vi "Take_photo.vi"(7 "error in":errorcluster, 10 "Session In":T3) -> (0 "error out":errorcluster, 2 "x = y?":bool)   [LabVIEW 2020]
doc: "Take photo if matching template."
uses:
  <vilib>/userDefined/High Color/IMAQdx.ctl
  <vilib>/vision/driver/NI_Vision_Acquisition_Software.lvlib
  <vilib>/vision/NI_Vision_Development_Module.lvlib
panel:
  out "Application Directory 3":path
  out "Application Directory 2":path
  out "Number of Matches":i32
  out "Image 2":T1(plugin-control)
  in  "Parameters":T2={"Number of Matches Requested"=1, "Minimum Match Score"=800.0, "Angle Ranges"=[]}
  out "Image":T1(plugin-control)
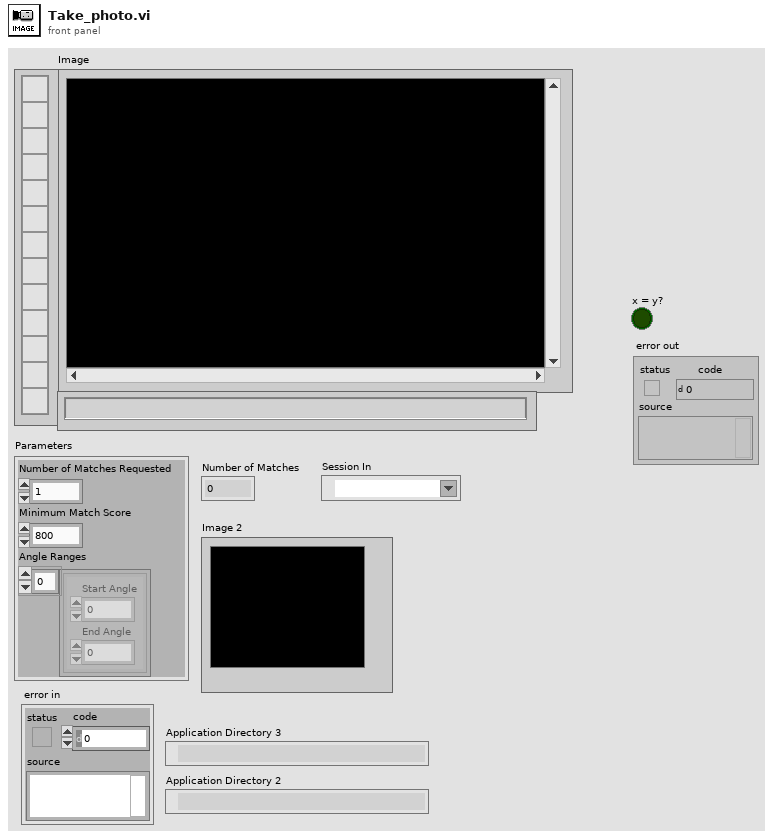
[diagram p1: front panel]
types:
  T1 = typedef "IMAQ Image.ctl" = refnum<image>
  T2 = cluster{"Number of Matches Requested":i32, "Minimum Match Score":sgl, "Angle Ranges":cluster{"Start Angle":sgl, "End Angle":sgl}[]}
  T3 = typedef "IMAQdx.ctl" = refnum<k21>
  T4 = cluster{"Position":cluster{"x":sgl, "y":sgl}, "Angle":sgl, "Scale":sgl, "Score":sgl, "Bounding Box":cluster{"x":sgl, "y":sgl}[]}[]
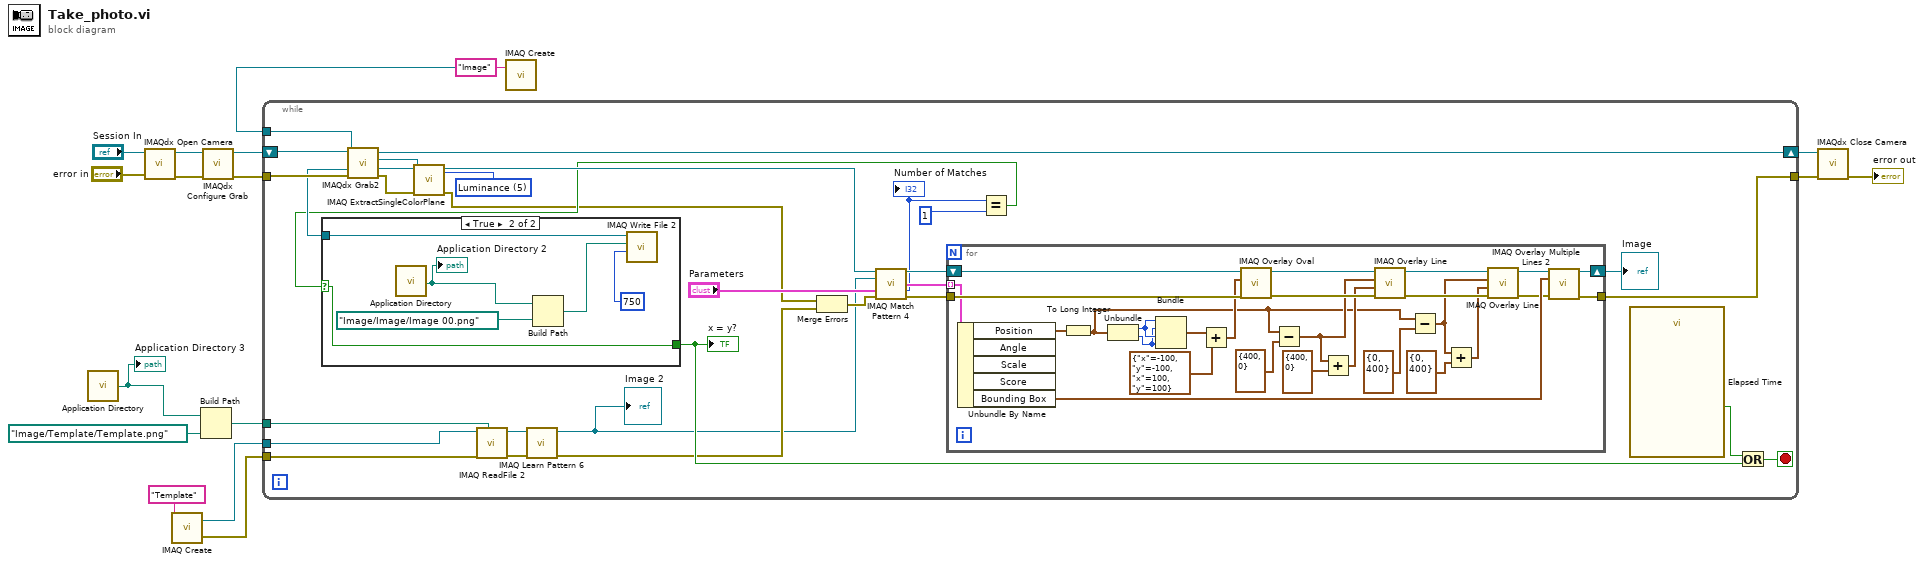
[diagram p0: block diagram]
diagram:
  n1 = call <vilib>:"Application Directory.vi"() -> ("Application Directory"=w4:path)
  "Application Directory 3" <- w4
  n2 = call <vilib>:"IMAQdx Open Camera.vi"("error in"="error in", "Session In"="Session In") -> ("error out"=w16:errorcluster, "Session Out"=w15:T3)  [unwired: 8 in]
  n3 = call "IMAQ Create"("Image Name"="Template") -> ("New Image"=w8:T1, "error out"=w7:errorcluster)  [unwired: 4 in]
  n4 = Build Path(base path=w4, name or relative path=path "Image/Template/Template.png") -> (appended path=w6:path)
  n5 = call <vilib>:"IMAQdx Configure Grab.vi"("error in"=w16, "Session In"=w15) -> ("error out"=w12:errorcluster, "Session Out"=w13:T3)  [unwired: 8 in]
  n6 = call "IMAQ Create"("Image Name"="Image") -> ("New Image"=w10:T1)  [unwired: 4 in, 1 out]
  n7 = while {
    tunnel: w12 -> [w46]
    shift-right: [w45] -> w11
    shift-left: w13 -> [w43]
    tunnel: w10 -> [w44]
    tunnel: w8 -> [w40]
    tunnel: w6 -> [w29]
    tunnel: w7 -> [w27]
    tunnel: [w19] -> w2
    stop <- w23 stop-if-true
    w42 = 5 items=["Red", "Green", "Blue", "Hue", "Saturation", "Luminance", "Value", "Intensity"] ("Color Plane")
    n8 = call <vilib>:"IMAQdx Grab2.vi"("error in"=w46, "Image In"=w44, "Session In"=w43) -> ("error out"=w28:errorcluster, "Image Out"=w41:T1, "Session Out"=w45:T3)  [unwired: 5 in, 1 out]
    n9 = call "IMAQ ExtractSingleColorPlane"("Color Plane"=w42, "error in (no error)"=w28, "Image Src"=w41) -> ("error out"=w22:errorcluster, "Image Dst Out"=w37:T1)  [unwired: 1 in, 6 out]
    n10 = call "IMAQ ReadFile 2"("File Path"=w29, "error in (no error)"=w27, "Image"=w40) -> ("error out"=w38:errorcluster, "Image Out"=w39:T1)  [unwired: 4 in, 3 out]
    n11 = call "IMAQ Learn Pattern 6"("Image"=w39, "error in (no error)"=w38) -> ("Template Image Out"=w18:T1, "error out"=w21:errorcluster)  [unwired: 11 in, 1 out]
    "Image 2" <- w18
    n12 = Merge Errors(w22, w21) -> (w20:errorcluster)
    n13 = call "IMAQ Match Pattern 4"("Image"=w37, "Template Image"=w18, "Parameters"="Parameters", "error in (no error)"=w20) -> ("Image (duplicate)"=w35:T1, "Matches (real-world)"=w32:T4, "Number of Matches"=w31:i32, "error out"=w33:errorcluster)  [unwired: 7 in, 1 out]
    "Number of Matches" <- w31
    n14 = for {
      tunnel: w33 -> [w68]
      tunnel: w32 -> [w65] mode=indexing
      shift-right: [w69] -> w34
      shift-left: w35 -> [w73]
      tunnel: [w49] -> w19
      n15 = Unbundle By Name(w65) -> ("Position"=w56:cluster{"x":sgl, "y":sgl}, "Bounding Box"=w62:cluster{"x":sgl, "y":sgl}[])  [unwired: 3 out]
      n16 = To Long Integer(number=w56) -> (32bit integer=w55:cluster{"x":i32, "y":i32})
      n17 = Unbundle(w55) -> ("x"=w64:i32, "y"=w63:i32)
      n18 = Bundle("x"=w64, "y"=w63, "x"=w64, "y"=w63) -> (w61:cluster{"x":i32, "y":i32, "x":i32, "y":i32})  [unwired: 1 in]
      n19 = Add(x=w61, y=cluster{"x":i32, "y":i32, "x":i32, "y":i32} {"x"=-100, "y"=-100, "x"=100, "y"=100}) -> (x+y=w60:cluster{"x":i32, "y":i32, "x":i32, "y":i32})
      n20 = call "IMAQ Overlay Oval"("error in (no error)"=w68, "Bounding Rectangle"=w60, "Image"=w73) -> ("error out"=w67:errorcluster, "Image Out"=w72:T1)  [unwired: 7 in]
      n21 = Subtract(x=w55, y=cluster{"x":i32, "y":i32} {"x"=400, "y"=0}) -> (x-y=w58:cluster{"x":i32, "y":i32})
      n22 = Add(x=w58, y=cluster{"x":i32, "y":i32} {"x"=400, "y"=0}) -> (x+y=w57:cluster{"x":i32, "y":i32})
      n23 = call "IMAQ Overlay Line"("error in (no error)"=w67, "End Point"=w57, "Start Point"=w58, "Image"=w72) -> ("error out"=w66:errorcluster, "Image Out"=w71:T1)  [unwired: 6 in]
      n24 = Subtract(x=w55, y=cluster{"x":i32, "y":i32} {"x"=0, "y"=400}) -> (x-y=w52:cluster{"x":i32, "y":i32})
      n25 = Add(x=w52, y=cluster{"x":i32, "y":i32} {"x"=0, "y"=400}) -> (x+y=w50:cluster{"x":i32, "y":i32})
      n26 = call "IMAQ Overlay Line"("error in (no error)"=w66, "End Point"=w50, "Start Point"=w52, "Image"=w71) -> ("error out"=w47:errorcluster, "Image Out"=w70:T1)  [unwired: 6 in]
      n27 = call "IMAQ Overlay Multiple Lines 2"("Image"=w70, "Line End Points"=w62, "error in (no error)"=w47) -> ("Image Out"=w69:T1, "error out"=w49:errorcluster)  [unwired: 11 in]
    }
    "Image" <- w34
    n28 = Equal?(x=w31, y=1) -> (x = y?=w26:bool)
    n29 = case shown="True" w26 {
      selector: w26 -> [w74 w78]
      tunnel: w37 -> [_ w79]
      tunnel: [w74 w78] -> w24
      frame False {
      }
      frame True {
        n30 = call <vilib>:"Application Directory.vi"() -> ("Application Directory"=w75:path)
        "Application Directory 2" <- w75
        n31 = Build Path(base path=w75, name or relative path=path "Image/Image/Image 00.png") -> (appended path=w77:path)
        n32 = call-poly "IMAQ Write File 2"("Image Quality"=u32 750, "File Path"=w77, "Image"=w79) -> ()  [unwired: 7 in, 2 out]
      }
    }
    "x = y?" <- w24
    n33 = call "Elapsed Time"() -> ("Time has Elapsed"=w25:bool)  [unwired: 12 in, 7 out]
    n34 = Or(x=w25, y=w24) -> (x .or. y?=w23:bool)
  }
  n35 = call <vilib>:"IMAQdx Close Camera.vi"("error in"=w2, "Session In"=w11) -> ("error out"=→"error out":errorcluster)  [unwired: 9 in]
